vi "NET_DriveRPM.vi"(8 "Read(F) Write(T)":bool, 11 "Drive Encoder Vel":T1) -> (3 "Drive RPM Out":T1)   [LabVIEW 2016]
uses:
  TypeDef/Cluster_Drive_RPM.ctl
  <vilib>/Rock Robotics/Network Tables/NT Write Numeric Array.vi
  <vilib>/Rock Robotics/Network Tables/NT Read Numeric Array.vi
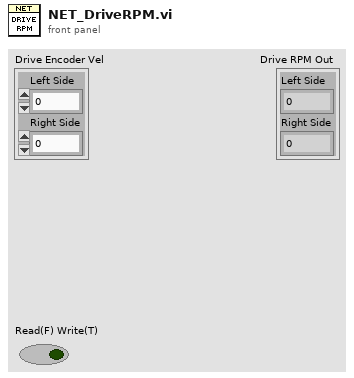
[diagram p1: front panel]
types:
  T1 = typedef "Cluster_Drive_RPM.ctl" = cluster{"Left Side":dbl, "Right Side":dbl}
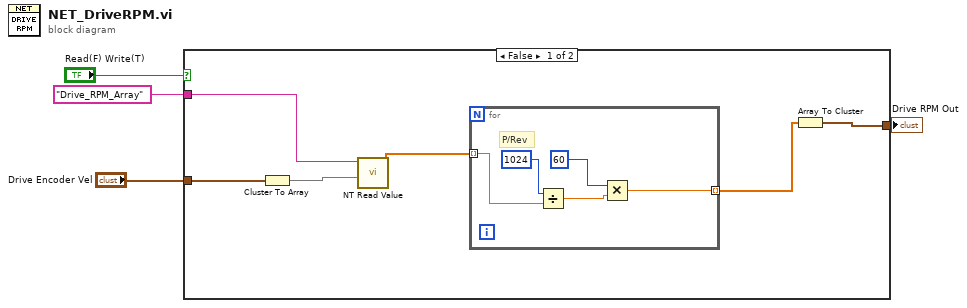
[diagram p0: block diagram]
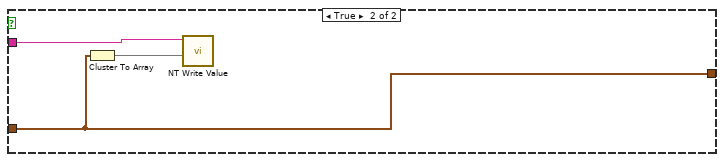
[diagram p2: hidden frame]
diagram:
  n1 = case shown="False" "Read(F) Write(T)" {
    tunnel: "Drive Encoder Vel" -> [w9 w16]
    tunnel: "Drive_RPM_Array" ("Name") -> [w10 w17]
    tunnel: [w7 w16] -> w1
    frame False {
      n2 = Cluster To Array(cluster=w9) -> (array=w8:dbl[])
      n3 = call-poly <vilib>:"NT Read Value.vi"("Default Value"=w8, "Name"=w10) -> ("Numeric Array"=w6:dbl[])  [unwired: 8 in, 1 out]
      n4 = for {
        tunnel: w6 -> [w12] mode=indexing
        tunnel: [w11] -> w5 mode=indexing
        # "P/Rev"
        n5 = Divide(x=1024, y=w12) -> (x/y=w13:dbl)
        n6 = Multiply(x=60, y=w13) -> (x*y=w11:dbl)
      }
      n7 = Array To Cluster(array=w5) -> (cluster=w7:cluster{"[0]":dbl, "[1]":dbl})
    }
    frame True {
      n8 = Cluster To Array(cluster=w16) -> (array=w18:dbl[])
      n9 = call-poly <vilib>:"NT Write Value.vi"("Numeric Array"=w18, "Name"=w17) -> ()  [unwired: 9 in, 1 out]
    }
  }
  "Drive RPM Out" <- w1
